vi "Serial_Communication.vi"() -> ()   [LabVIEW 2023]
uses:
  <vilib>/Instr/_visa.llb/VISA Configure Serial Port (Instr).vi
panel:
  out "Present Time":string caption="Present Text"
  out "error in (no error)":errorcluster
  in  "Tab Control":enum32{"Page 1", "Page 2"}(tab)
  out "Waveform Chart - Dark":cluster{"Meter":dbl, "Gauge":dbl}(graph)
  in  "Clear":bool
  out "Meter":dbl(knob) caption="Gauge" scale=0.0..500.0
  out "Gauge":dbl(knob) scale=0.0..500.0
  in  "Loop Status":bool
  in  "Send Button":bool
  in  "Send Data":string
  out "Data Received":string
  in  "COM Port":refnum<visa-resource-name>
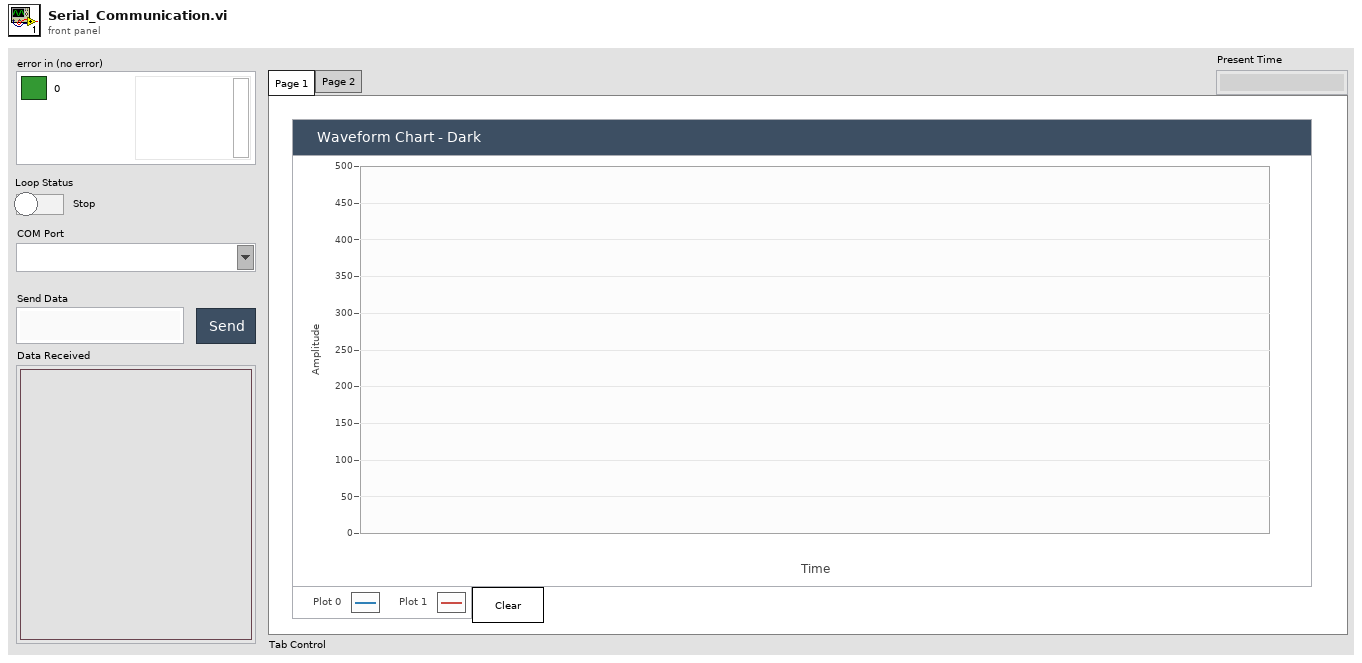
[diagram p1: front panel]
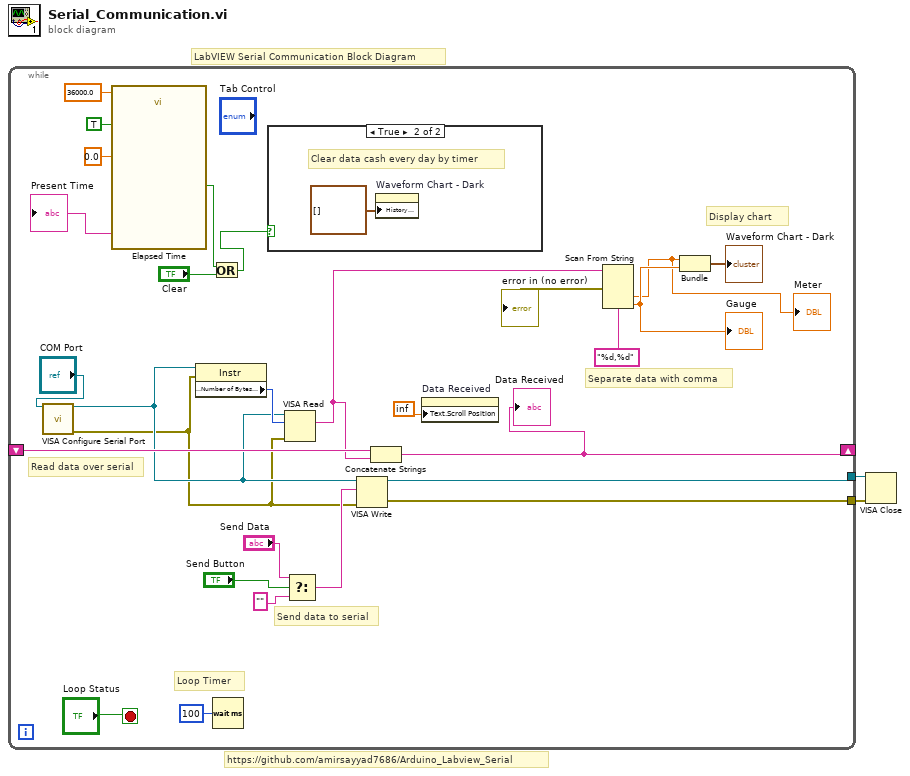
[diagram p0: block diagram]
diagram:
  # "https://github.com/amirsayyad7686/Arduino_Labview_Serial"
  # "LabVIEW Serial Communication Block Diagram"
  n1 = while {
    tunnel: [w19] -> w2
    tunnel: [w18] -> w1
    shift-right: [w6] -> _
    shift-left: _ -> [w29]
    stop <- "Loop Status" stop-if-true
    # "Separate data with comma"
    # "Display chart"
    # "Loop Timer"
    # "Send data to serial"
    # "Read data over serial"
    n2 = call-poly "VISA Configure Serial Port"("VISA resource name"="COM Port") -> ("VISA resource name out"=w16:refnum<visa-resource-name>, "error out"=w15:errorcluster)  [unwired: 13 in]
    n3 = call "Elapsed Time"("Time Target (s)"=36000.0, "Auto Reset"=TRUE, "Set Start Time (s)"=0.0) -> ("Present Text"=→"Present Time":string, "Time has Elapsed"=w10:bool)  [unwired: 9 in, 6 out]
    n4 = property class="Instr"(reference=w16, error in=w15) -> ("Serial Settings:Number of Bytes at Serial Port"=w30:u32)  [unwired: 2 out]
    n5 = Or(x=w10, y="Clear") -> (x .or. y?=w8:bool)
    n6 = Wait (ms)(milliseconds to wait=u32 100) -> ()  [unwired: 1 out]
    n7 = case shown="True" w8 {
      frame False {
      }
      frame True {
        # "Clear data cash every day by timer"
        n8 = property on="Waveform Chart - Dark" class="WFChart (strict)"("History Data"=cluster{i32, "Waveform Chart":dbl}[] []) -> ()  [unwired: 2 in, 2 out]
      }
    }
    n9 = VISA Read(VISA resource name=w16, byte count=w30, error in (no error)=w15) -> (read buffer=w22:string)  [unwired: 3 out]
    n10 = Select(t="Send Data", s="Send Button", f="") -> (s? t:f=w26:string)
    n11 = VISA Write(VISA resource name=w16, write buffer=w26, error in (no error)=w15) -> (VISA resource name out=w19:refnum<visa-resource-name>, error out=w18:errorcluster)  [unwired: 1 out]
    n12 = Concatenate Strings(w29, w22) -> (w6:string)
    "Data Received" <- w6
    n13 = property on="Data Received" class="Str"("Text.Scroll Position"=inf) -> ()  [unwired: 2 in, 2 out]
    n14 = Scan From String(format string="%d,%d", input string=w22) -> (error out=→"error in (no error)":errorcluster, output 1=w3:dbl, output 2=w4:dbl)  [unwired: 4 in, 2 out]
    "Meter" <- w3
    "Gauge" <- w4
    n15 = Bundle("Meter"=w3, "Gauge"=w4) -> (→"Waveform Chart - Dark":cluster{"Meter":dbl, "Gauge":dbl})  [unwired: 1 in]
  }
  n16 = VISA Close(VISA resource name=w2, error in (no error)=w1) -> ()  [unwired: 1 out]
